vi "读取模拟数据子程序.vi"() -> (0 "Input":T1={"Digital Start Trigger Source 4"="/Dev1/PFI0", "Digital Start Trigger Edge 4"=10280, "minimum value"=-10.0, "maximum value"=10.0, "rate"=1000.0, "device name"="PXI1Slot5", "formular in"=[], "Total time"=0.0} {"rate" format="%0.2f"; "maximum value" format="%0.2f"; "minimum value" format="%0.2f"; "Digital Start Trigger Edge 4" items=["Rising"=10280, "Falling"=10171]})   [LabVIEW 2021]
uses:
  <vilib>/Utility/file.llb/Read Delimited Spreadsheet (string).vi
panel:
  # "1、formular in 中sample为各个分段函数的持续时间。\n2、Total time 为总时间，必须大于sample加起来的值。\n3、minimum value和maximum value默认±10V不改。\n4、rate为采样率，即时钟频率\n5、device name为选择的板卡名字，可选为PXI1Slot5-7\n6、Source 为接受触发的端口，Edge为选择上升沿触发\n还是其他类型触发。"
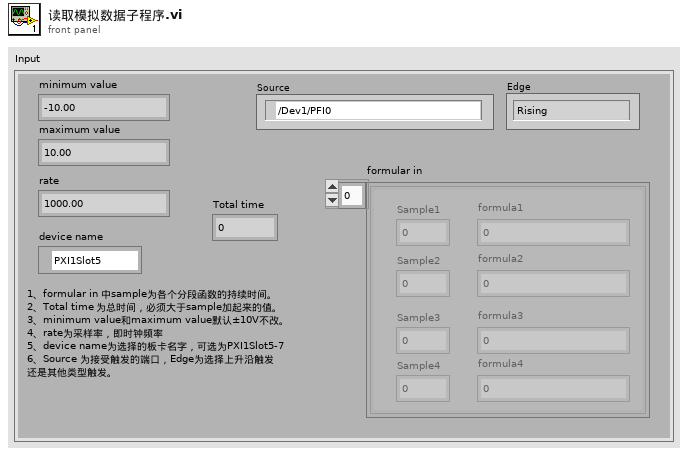
[diagram p1: front panel]
types:
  T1 = cluster{"Digital Start Trigger Source 4":tag, "Digital Start Trigger Edge 4":i32, "minimum value":dbl, "maximum value":dbl, "rate":dbl, "device name":tag, "formular in":cluster{"Sample1":dbl, "formula1":string, "Sample2":dbl, "formula2":string, "Sample3":dbl, "formula3":string, "Sample4":dbl, "formula4":string}[], "Total time":dbl}
  T2 = cluster{"Sample1":dbl, "formula1":string, "Sample2":dbl, "formula2":string, "Sample3":dbl, "formula3":string, "Sample4":dbl, "formula4":string}
  T3 = cluster{"all rows[0]":string, "all rows[1]":string, "all rows[2]":string, "all rows[3]":string, "all rows[4]":string, "all rows[5]":string, "all rows[6]":string, "all rows[7]":string, "all rows[8]":string}
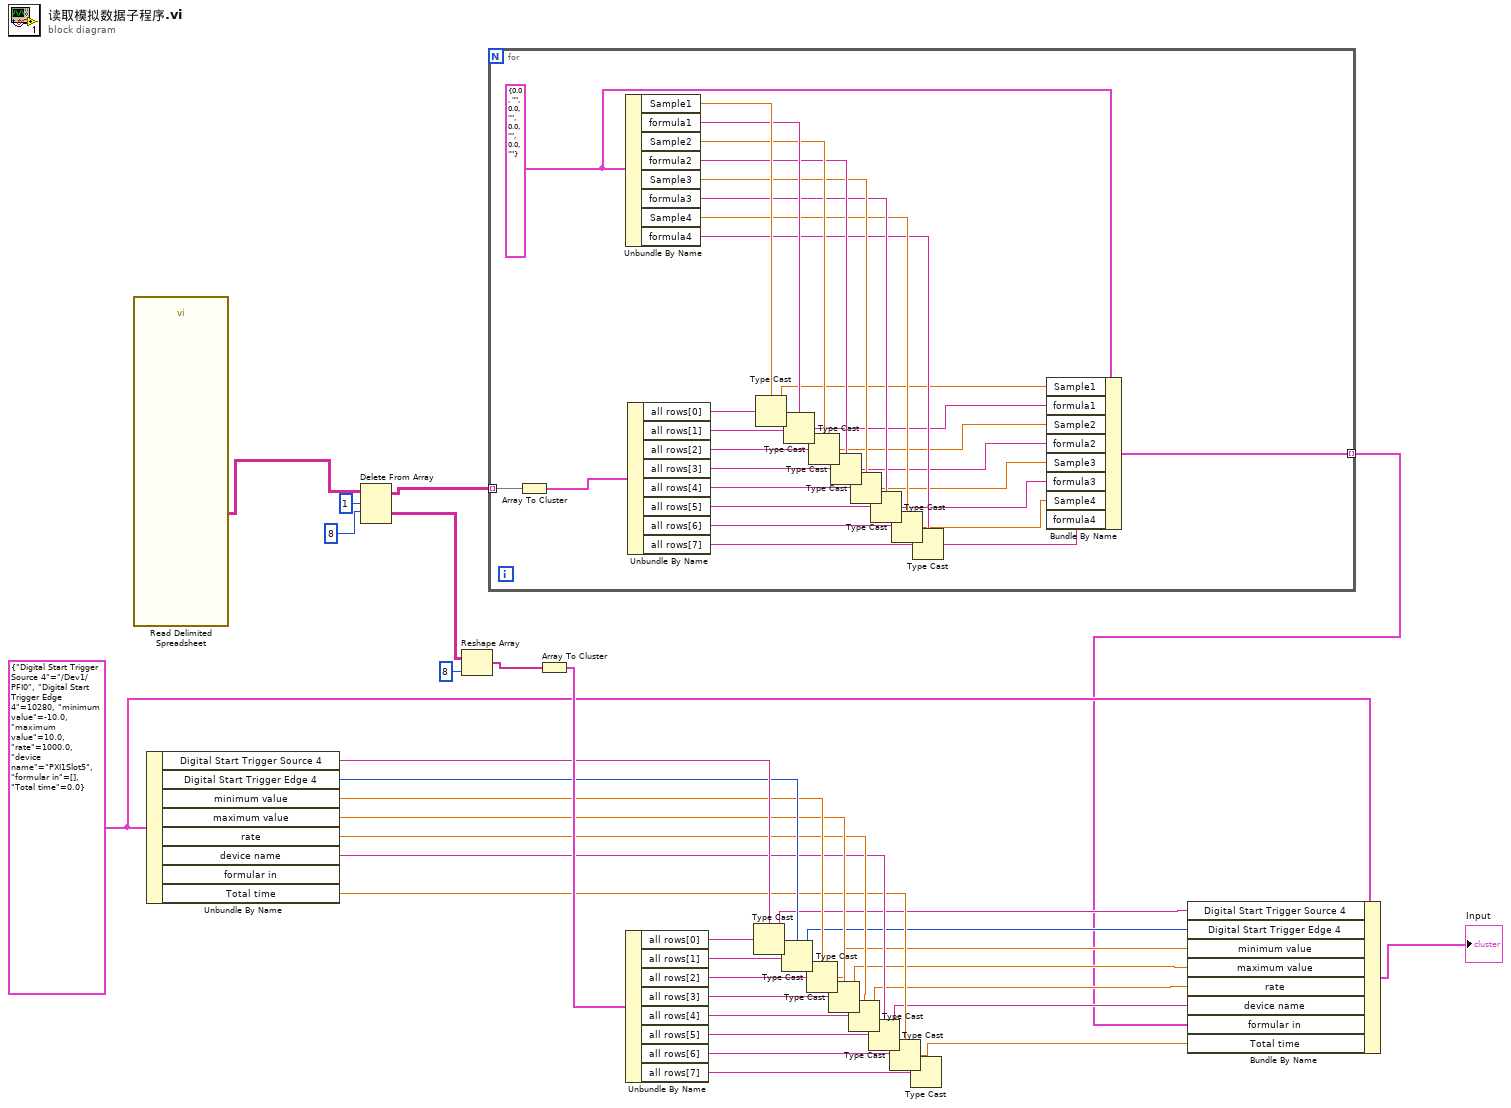
[diagram p0: block diagram]
diagram:
  w10 = T1 {"Digital Start Trigger Source 4"="/Dev1/PFI0", "Digital Start Trigger Edge 4"=10280, "minimum value"=-10.0, "maximum value"=10.0, "rate"=1000.0, "device name"="PXI1Slot5", "formular in"=[], "Total time"=0.0} ("Input")
  n1 = call-poly <vilib>:"Read Delimited Spreadsheet.vi"() -> ("all rows"=w30:string[][])  [unwired: 10 in, 5 out]
  n2 = Unbundle By Name(w10) -> ("Digital Start Trigger Source 4"=w17:tag, "Digital Start Trigger Edge 4"=w16:i32, "minimum value"=w15:dbl, "maximum value"=w14:dbl, "rate"=w13:dbl, "device name"=w12:tag, "Total time"=w11:dbl)  [unwired: 1 out]
  n3 = Delete From Array(array=w30, length=1, index (row)=8) -> (deleted portion=w29:string[][], array with subset deleted=w31:string[][])  [unwired: 1 in]
  n4 = Reshape Array(w29, 8 ("dimension size")) -> (w27:string[])
  n5 = for {
    tunnel: w31 -> [w61] mode=indexing
    tunnel: [w34] -> w2 mode=indexing
    w43 = T2 {"Sample1"=0.0, "formula1"="", "Sample2"=0.0, "formula2"="", "Sample3"=0.0, "formula3"="", "Sample4"=0.0, "formula4"=""} ("formular in[0]")
    n6 = Array To Cluster(array=w61) -> (cluster=w60:T3)
    n7 = Unbundle By Name(w43) -> ("Sample1"=w58:dbl, "formula1"=w57:string, "Sample2"=w54:dbl, "formula2"=w52:string, "Sample3"=w50:dbl, "formula3"=w48:string, "Sample4"=w46:dbl, "formula4"=w44:string)
    n8 = Unbundle By Name(w60) -> ("all rows[0]"=w59:string, "all rows[1]"=w56:string, "all rows[2]"=w55:string, "all rows[3]"=w53:string, "all rows[4]"=w51:string, "all rows[5]"=w49:string, "all rows[6]"=w47:string, "all rows[7]"=w45:string)
    n9 = Type Cast(type=w58, x=w59) -> (*(type *) &x=w42:dbl)
    n10 = Type Cast(type=w57, x=w56) -> (*(type *) &x=w41:string)
    n11 = Type Cast(type=w54, x=w55) -> (*(type *) &x=w40:dbl)
    n12 = Type Cast(type=w52, x=w53) -> (*(type *) &x=w39:string)
    n13 = Type Cast(type=w50, x=w51) -> (*(type *) &x=w38:dbl)
    n14 = Type Cast(type=w48, x=w49) -> (*(type *) &x=w37:string)
    n15 = Type Cast(type=w46, x=w47) -> (*(type *) &x=w36:dbl)
    n16 = Type Cast(type=w44, x=w45) -> (*(type *) &x=w35:string)
    n17 = Bundle By Name(cluster=w43, "Sample1"=w42, "formula1"=w41, "Sample2"=w40, "formula2"=w39, "Sample3"=w38, "formula3"=w37, "Sample4"=w36, "formula4"=w35) -> (w34:T2)
  }
  n18 = Array To Cluster(array=w27) -> (cluster=w18:T3)
  n19 = Unbundle By Name(w18) -> ("all rows[0]"=w26:string, "all rows[1]"=w25:string, "all rows[2]"=w24:string, "all rows[3]"=w23:string, "all rows[4]"=w22:string, "all rows[5]"=w21:string, "all rows[6]"=w20:string, "all rows[7]"=w19:string)
  n20 = Type Cast(type=w17, x=w26) -> (*(type *) &x=w9:tag)
  n21 = Type Cast(type=w16, x=w25) -> (*(type *) &x=w8:i32)
  n22 = Type Cast(type=w15, x=w24) -> (*(type *) &x=w7:dbl)
  n23 = Type Cast(type=w14, x=w23) -> (*(type *) &x=w6:dbl)
  n24 = Type Cast(type=w13, x=w22) -> (*(type *) &x=w5:dbl)
  n25 = Type Cast(type=w12, x=w21) -> (*(type *) &x=w4:tag)
  n26 = Type Cast(type=w11, x=w20) -> (*(type *) &x=w3:dbl)
  n27 = Type Cast(x=w19) -> ()  [unwired: 1 in, 1 out]
  n28 = Bundle By Name(cluster=w10, "Digital Start Trigger Source 4"=w9, "Digital Start Trigger Edge 4"=w8, "minimum value"=w7, "maximum value"=w6, "rate"=w5, "device name"=w4, "formular in"=w2, "Total time"=w3) -> (→"Input":T1)
